vi "XDataNode8_5To8_2.vi"(10 "Version-State Cluster In":T1, 11 "XRef":refnum<vi>) -> (0 "Custom Label":string, 1 "Custom Warning To Issue":string, 2 "Version-State Cluster Out":T1, 3 "Action":T2)   [LabVIEW 2017]
uses:
  <vilib>/XSFPSupport/SFPChangeStateAction.ctl
  <vilib>/XNodeSupport/XNodeVersion.ctl
  <vilib>/XNodeSupport/XNodeUShort.ctl
  <vilib>/Platform/TimedLoop/XDataNode/XDataNode8_5_0_1.ctl
  <vilib>/Platform/TimedLoop/XDataNode/nitl_modes.ctl
  <vilib>/Platform/TimedLoop/XDataNode/wakeup.ctl
  <vilib>/Platform/TimedLoop/XDataNode/TermInfo.ctl
  <vilib>/Platform/TimedLoop/XDataNode/nitl_TargetSpecificData.ctl
  <vilib>/Platform/TimedLoop/XDataNode/DN_Type.ctl
  <vilib>/Platform/TimedLoop/XDataNode/XDataNode8_0_6_3.ctl
  <vilib>/XSFPSupport/NI_XSFPSupport.lvlib
  <vilib>/XNodeSupport/NI_XNodeSupport.lvlib
  <vilib>/Platform/TimedLoop/XDataNode/XDataNode.xnode
  <vilib>/Platform/TimedLoop/XDataNode/XDNodeRunTimeDep.lvlib
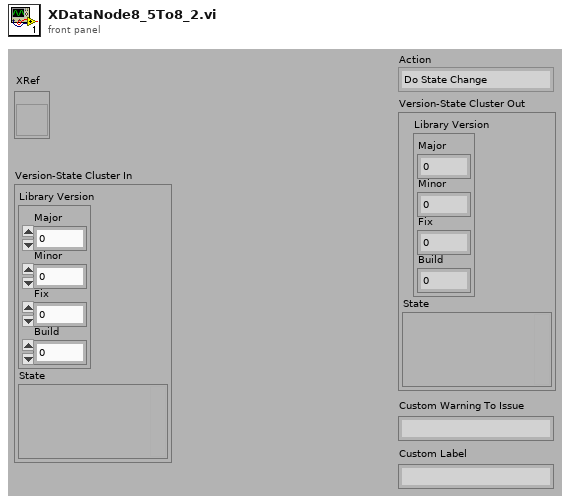
[diagram p1: front panel]
types:
  T1 = cluster{"Library Version":cluster{"Major":u16, "Minor":u16, "Fix":u16, "Build":u16}, "State":variant}
  T2 = typedef "NI_XSFPSupport.lvlib/SFPChangeStateAction.ctl" = enum32{"Do State Change", "Replace With Label", "Fail SFP"}
  T3 = typedef "NI_XNodeSupport.lvlib/XNodeVersion.ctl" = cluster{"Major":T4, "Minor":T4, "Fix":T4, "Build":T4}
  T4 = typedef "NI_XNodeSupport.lvlib/XNodeUShort.ctl" = u16
  T5 = typedef "XDataNode.xnode/XDataNode8_0_6_3.ctl" = cluster{"Timing":cluster{"Expected End [f-1]":u64, "Actual End [f-1]":u64, "Finished Late? [f-1]":bool, "Expected End [i-1]":u64, "Actual End [i-1]":u64, "Finished Late? [i-1]":bool, "Expected Start [i]":u64, "Actual Start [i]":u64, "Expected Start [f]":u64, "Actual Start [f]":u64, "Source Name":string, "Name":string, "Period":i64, "Deadline":i64, "Offset":i64, "Start":i64, "Priority":i32, "Timeout":i32, "Mode":T6, "Wakeup Reason":T7, "Error":errorcluster, "Source Type":string, "Secondary Source Type":string, "Global End Time":u64, "Global Start Time":u64, "Frame Duration":u64, "Iteration Duration":u64}, "Size":T8[], "Hidden":T8[], "Invisible":bool[], "Input?":bool, "timing src wired?":bool, "Target Specific Data":T9[], "G Only Data":variant, "DataNode_Type":enum32{"TL_Lft_Ear", "TL_Rt_Ear", "TL_Lft_Dn", "TL_Rf_Dn", "TS_Lft_Ear", "TS_Rt_Ear", "TS_1stFrame_Lft_Dn", "TS_Lft_Dn", "TS_LastFrame_Rt_Dn", "TS_Rt_Dn", "TL_TS_Lft_Ear", "TL_TS_Rt_Ear", "TL_TS_Lft_Dn", "TL_TS_Rt_Dn", "TL_TS_1stFrame_Lft_Dn", "TL_TS_LastFrame_Rt_Dn"}}
  T6 = typedef "XDNodeRunTimeDep.lvlib/nitl_modes.ctl" = enum32{"No Change", "Process missed periods, maintain original phase", "Discard missed periods, maintain original phase", "Process missed periods, ignore original phase", "Discard missed periods, ignore original phase"}
  T7 = typedef "XDNodeRunTimeDep.lvlib/wakeup.ctl" = enum32{"Normal", "Aborted", "Asynchronous wakeup", "Timing source error", "Timed loop error", "Timeout"}
  T8 = typedef "XDataNode.xnode/TermInfo.ctl" = cluster{"ID":i32, "Wired?":bool, "Type":variant, "Name":string, "Input?":bool, "StaticID":i32}
  T9 = typedef "XDataNode.xnode/nitl_TargetSpecificData.ctl" = cluster{"Target Name":string, "Target Data":variant}
  T10 = typedef "XDataNode.xnode/XDataNode8_5_0_1.ctl" = cluster{"Timing":cluster{"Expected End [f-1]":u64, "Actual End [f-1]":u64, "Finished Late? [f-1]":bool, "Expected End [i-1]":u64, "Actual End [i-1]":u64, "Finished Late? [i-1]":bool, "Expected Start [i]":u64, "Actual Start [i]":u64, "Expected Start [f]":u64, "Actual Start [f]":u64, "Source Name":string, "Name":string, "Period":i64, "Deadline":i64, "Offset":i64, "Start":i64, "Priority":i32, "Timeout":i32, "Mode":T6, "Wakeup Reason":T7, "Error":errorcluster, "Source Type":string, "Secondary Source Type":string, "Global End Time":u64, "Global Start Time":u64, "Frame Duration":u64, "Iteration Duration":u64, "Assigned CPU":i32}, "Size":T8[], "Hidden":T8[], "Invisible":bool[], "Input?":bool, "timing src wired?":bool, "Target Specific Data":T9[], "G Only Data":variant, "DataNode_Type":T11}
  T11 = typedef "XDataNode.xnode/DN_Type.ctl" = enum32{"TL_Lft_Ear", "TL_Rt_Ear", "TL_Lft_Dn", "TL_Rt_Dn", "TS_Lft_Ear", "TS_Rt_Ear", "TS_1stFrame_Lft_Dn", "TS_Lft_Dn", "TS_LastFrame_Rt_Dn", "TS_Rt_Dn", "TL_TS_Lft_Ear", "TL_TS_Rt_Ear", "TL_TS_Lft_Dn", "TL_TS_Rt_Dn", "TL_TS_1stFrame_Lft_Dn", "TL_TS_LastFrame_Rt_Dn"}
  T12 = cluster{"Major":u16, "Minor":u16, "Fix":u16, "Build":u16}
  T13 = cluster{"Expected End [f-1]":u64, "Actual End [f-1]":u64, "Finished Late? [f-1]":bool, "Expected End [i-1]":u64, "Actual End [i-1]":u64, "Finished Late? [i-1]":bool, "Expected Start [i]":u64, "Actual Start [i]":u64, "Expected Start [f]":u64, "Actual Start [f]":u64, "Source Name":string, "Name":string, "Period":i64, "Deadline":i64, "Offset":i64, "Start":i64, "Priority":i32, "Timeout":i32, "Mode":T6, "Wakeup Reason":T7, "Error":errorcluster, "Source Type":string, "Secondary Source Type":string, "Global End Time":u64, "Global Start Time":u64, "Frame Duration":u64, "Iteration Duration":u64, "Assigned CPU":i32}
  T14 = cluster{"Expected End [f-1]":u64, "Actual End [f-1]":u64, "Finished Late? [f-1]":bool, "Expected End [i-1]":u64, "Actual End [i-1]":u64, "Finished Late? [i-1]":bool, "Expected Start [i]":u64, "Actual Start [i]":u64, "Expected Start [f]":u64, "Actual Start [f]":u64, "Source Name":string, "Name":string, "Period":i64, "Deadline":i64, "Offset":i64, "Start":i64, "Priority":i32, "Timeout":i32, "Mode":T6, "Wakeup Reason":T7, "Error":errorcluster, "Source Type":string, "Secondary Source Type":string, "Global End Time":u64, "Global Start Time":u64, "Frame Duration":u64, "Iteration Duration":u64}
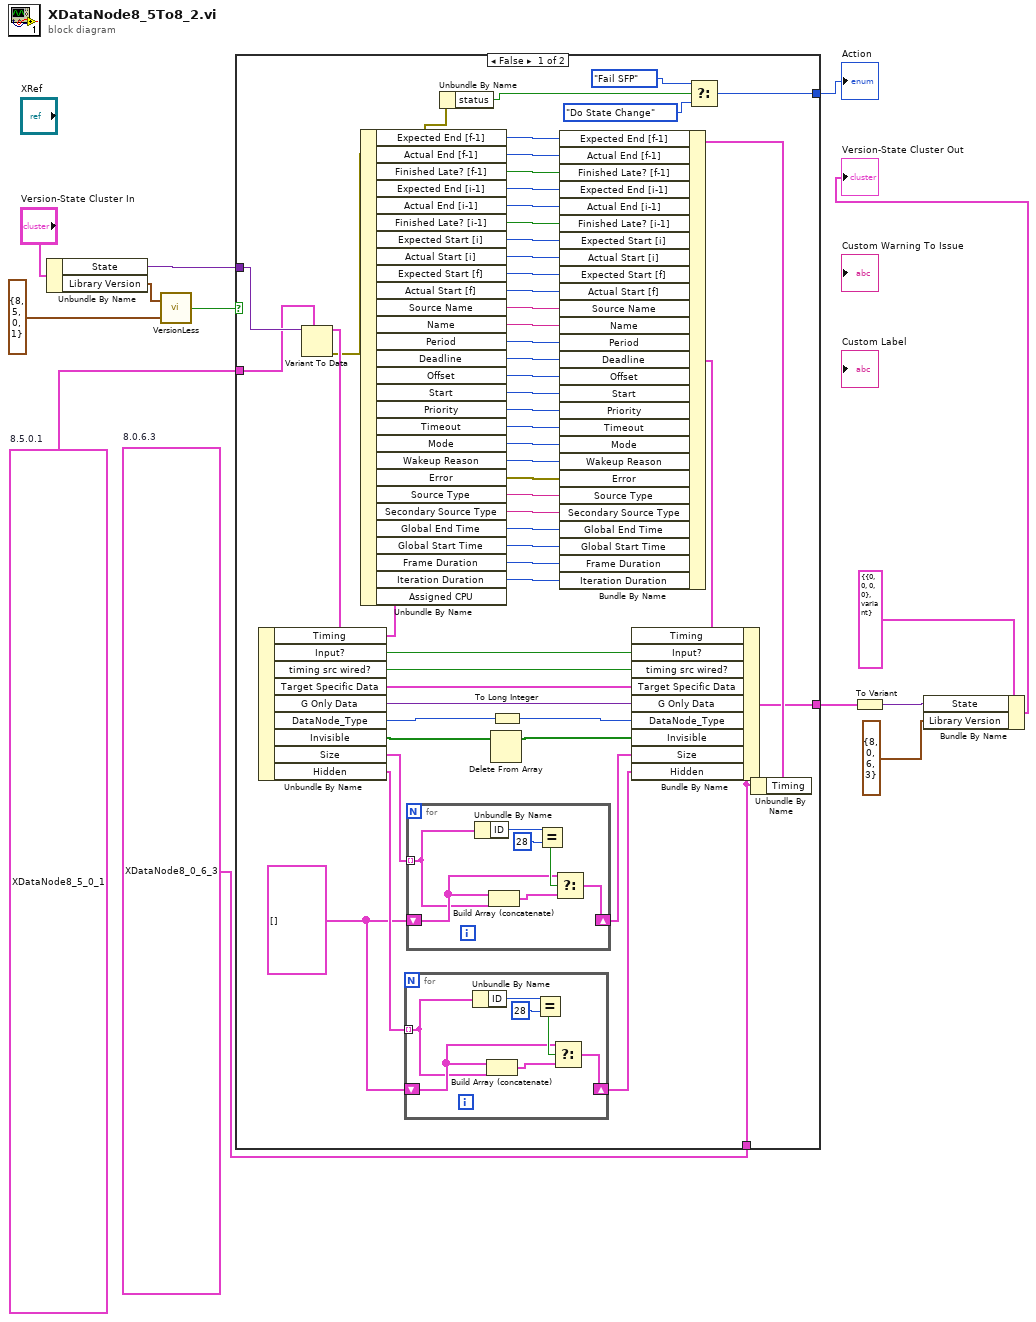
[diagram p0: block diagram]
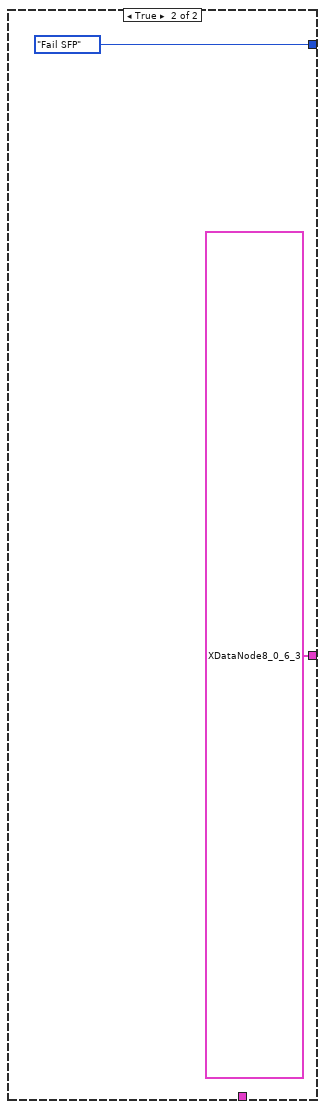
[diagram p2: hidden frame]
diagram:
  w6 = T5 {"Timing"={"Expected End [f-1]"=0, "Actual End [f-1]"=0, "Finished Late? [f-1]"=FALSE, "Expected End [i-1]"=0, "Actual End [i-1]"=0, "Finished Late? [i-1]"=FALSE, "Expected Start [i]"=0, "Actual Start [i]"=0, "Expected Start [f]"=0, "Actual Start [f]"=0, "Source Name"="", "Name"="", "Period"=0, "Deadline"=0, "Offset"=0, "Start"=0, "Priority"=0, "Timeout"=0, "Mode"=enum."No Change", "Wakeup Reason"=enum."Normal", "Error"={"status"=FALSE, "code"=0, "source"=""}, "Source Type"="", "Secondary Source Type"="", "Global End Time"=0, "Global Start Time"=0, "Frame Duration"=0, "Iteration Duration"=0}, "Size"=[], "Hidden"=[], "Invisible"=[], "Input?"=FALSE, "timing src wired?"=FALSE, "Target Specific Data"=[], "G Only Data"=variant, "DataNode_Type"=enum."TL_Lft_Ear"}  # 8.0.6.3
  w7 = T10 {"Timing"={"Expected End [f-1]"=0, "Actual End [f-1]"=0, "Finished Late? [f-1]"=FALSE, "Expected End [i-1]"=0, "Actual End [i-1]"=0, "Finished Late? [i-1]"=FALSE, "Expected Start [i]"=0, "Actual Start [i]"=0, "Expected Start [f]"=0, "Actual Start [f]"=0, "Source Name"="", "Name"="", "Period"=0, "Deadline"=0, "Offset"=0, "Start"=0, "Priority"=0, "Timeout"=0, "Mode"=enum."No Change", "Wakeup Reason"=enum."Normal", "Error"={"status"=FALSE, "code"=0, "source"=""}, "Source Type"="", "Secondary Source Type"="", "Global End Time"=0, "Global Start Time"=0, "Frame Duration"=0, "Iteration Duration"=0, "Assigned CPU"=0}, "Size"=[], "Hidden"=[], "Invisible"=[], "Input?"=FALSE, "timing src wired?"=FALSE, "Target Specific Data"=[], "G Only Data"=variant, "DataNode_Type"=enum."TL_Lft_Ear"}  # 8.5.0.1
  n1 = Unbundle By Name("Version-State Cluster In") -> ("State"=w8:variant, "Library Version"=w9:T12)
  n2 = call <vilib>:"VersionLess.vi"("y"=T3 {"Major"=8, "Minor"=5, "Fix"=0, "Build"=1}, "x"=w9) -> ("x < y?"=w11:bool)
  n3 = case shown="False" w11 {
    tunnel: [w15 SFPChangeStateAction."Fail SFP" ("Action")] -> w10
    tunnel: w8 -> [w66 _]
    tunnel: w7 -> [w65 _]
    tunnel: w6 -> [w62 _]
    tunnel: [w14 T5 {"Timing"={"Expected End [f-1]"=0, "Actual End [f-1]"=0, "Finished Late? [f-1]"=FALSE, "Expected End [i-1]"=0, "Actual End [i-1]"=0, "Finished Late? [i-1]"=FALSE, "Expected Start [i]"=0, "Actual Start [i]"=0, "Expected Start [f]"=0, "Actual Start [f]"=0, "Source Name"="", "Name"="", "Period"=0, "Deadline"=0, "Offset"=0, "Start"=0, "Priority"=0, "Timeout"=0, "Mode"=enum."No Change", "Wakeup Reason"=enum."Normal", "Error"={"status"=FALSE, "code"=0, "source"=""}, "Source Type"="", "Secondary Source Type"="", "Global End Time"=0, "Global Start Time"=0, "Frame Duration"=0, "Iteration Duration"=0}, "Size"=[], "Hidden"=[], "Invisible"=[], "Input?"=FALSE, "timing src wired?"=FALSE, "Target Specific Data"=[], "G Only Data"=variant, "DataNode_Type"=enum."TL_Lft_Ear"} ("8.0.6.3")] -> w5
    frame False {
      w20 = T8[] [] ("Size")
      n4 = Variant To Data(type=w65, Variant=w66) -> (data=w64:T10, error out=w19:errorcluster)  [unwired: 1 in]
      n5 = Unbundle By Name(w64) -> ("Timing"=w63:T13, "Input?"=w32:bool, "timing src wired?"=w31:bool, "Target Specific Data"=w30:T9[], "G Only Data"=w29:variant, "DataNode_Type"=w28:T11, "Invisible"=w26:bool[], "Size"=w24:T8[], "Hidden"=w22:T8[])
      n6 = Unbundle By Name(w63) -> ("Expected End [f-1]"=w60:u64, "Actual End [f-1]"=w59:u64, "Finished Late? [f-1]"=w58:bool, "Expected End [i-1]"=w57:u64, "Actual End [i-1]"=w56:u64, "Finished Late? [i-1]"=w55:bool, "Expected Start [i]"=w54:u64, "Actual Start [i]"=w53:u64, "Expected Start [f]"=w52:u64, "Actual Start [f]"=w51:u64, "Source Name"=w50:string, "Name"=w49:string, "Period"=w48:i64, "Deadline"=w47:i64, "Offset"=w46:i64, "Start"=w45:i64, "Priority"=w44:i32, "Timeout"=w43:i32, "Mode"=w42:T6, "Wakeup Reason"=w41:T7, "Error"=w40:errorcluster, "Source Type"=w39:string, "Secondary Source Type"=w38:string, "Global End Time"=w37:u64, "Global Start Time"=w36:u64, "Frame Duration"=w35:u64, "Iteration Duration"=w34:u64)  [unwired: 1 out]
      n7 = for {
        tunnel: w22 -> [w69] mode=indexing
        shift-right: [w67] -> w21
        shift-left: w20 -> [w70]
        n8 = Unbundle By Name(w69) -> ("ID"=w73:i32)
        n9 = Build Array (concatenate)(w70, w69) -> (w68:T8[])
        n10 = Equal?(x=w73, y=28) -> (x = y?=w71:bool)
        n11 = Select(t=w70, s=w71, f=w68) -> (s? t:f=w67:T8[])
      }
      n12 = for {
        tunnel: w24 -> [w76] mode=indexing
        shift-right: [w74] -> w23
        shift-left: w20 -> [w77]
        n13 = Unbundle By Name(w76) -> ("ID"=w80:i32)
        n14 = Build Array (concatenate)(w77, w76) -> (w75:T8[])
        n15 = Equal?(x=w80, y=28) -> (x = y?=w78:bool)
        n16 = Select(t=w77, s=w78, f=w75) -> (s? t:f=w74:T8[])
      }
      n17 = Unbundle By Name(w19) -> ("status"=w18:bool)
      n18 = Delete From Array(array=w26) -> (array with subset deleted=w25:bool[])  [unwired: 2 in, 1 out]
      n19 = To Long Integer(number=w28) -> (32bit integer=w27:i32)
      n20 = Select(t=SFPChangeStateAction."Fail SFP" ("Action"), s=w18, f=SFPChangeStateAction."Do State Change" ("Action")) -> (s? t:f=w15:T2)
      n21 = Unbundle By Name(w62) -> ("Timing"=w61:T14)
      n22 = Bundle By Name(cluster=w61, "Expected End [f-1]"=w60, "Actual End [f-1]"=w59, "Finished Late? [f-1]"=w58, "Expected End [i-1]"=w57, "Actual End [i-1]"=w56, "Finished Late? [i-1]"=w55, "Expected Start [i]"=w54, "Actual Start [i]"=w53, "Expected Start [f]"=w52, "Actual Start [f]"=w51, "Source Name"=w50, "Name"=w49, "Period"=w48, "Deadline"=w47, "Offset"=w46, "Start"=w45, "Priority"=w44, "Timeout"=w43, "Mode"=w42, "Wakeup Reason"=w41, "Error"=w40, "Source Type"=w39, "Secondary Source Type"=w38, "Global End Time"=w37, "Global Start Time"=w36, "Frame Duration"=w35, "Iteration Duration"=w34) -> (w33:T14)
      n23 = Bundle By Name(cluster=w62, "Timing"=w33, "Input?"=w32, "timing src wired?"=w31, "Target Specific Data"=w30, "G Only Data"=w29, "DataNode_Type"=w27, "Invisible"=w25, "Size"=w23, "Hidden"=w21) -> (w14:T5)
    }
    frame True {
    }
  }
  "Action" <- w10
  n24 = To Variant(anything=w5) -> (Variant=w4:variant)
  n25 = Bundle By Name(cluster=T1 {"Library Version"={"Major"=0, "Minor"=0, "Fix"=0, "Build"=0}, "State"=variant} ("Version-State Cluster Out"), "State"=w4, "Library Version"=T3 {"Major"=8, "Minor"=0, "Fix"=6, "Build"=3} ("y")) -> (→"Version-State Cluster Out":T1)
